vi "LogBuffer.vi"(0 "tdms file in":refnum<k34>, 1 "Buffer in":refnum<queue>, 5 "sizeOfBlock":i32, 7 "NumOfChannels":i32=65, 11 "error in (no error)":errorcluster, 12 "resetResample":bool, 13 "resample factor":cluster{"interpolation":i32, "decimation":i32}={"interpolation"=1, "decimation"=25}) -> (4 "tdms file out":refnum<k34>, 15 "error out":errorcluster)   [LabVIEW 2017, in "BufferLogging.lvlib"]
doc: "Log a single buffer. Decimate if configured."
uses:
  BufferLogging.lvlib
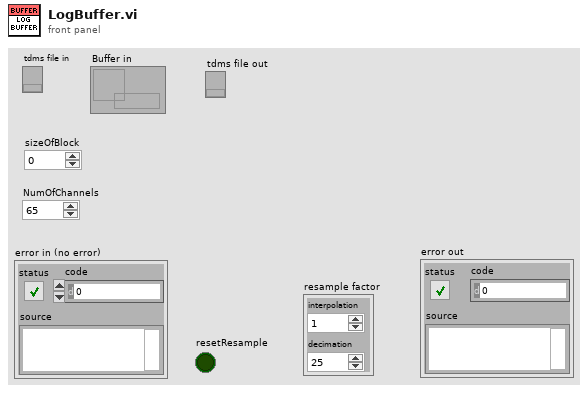
[diagram p1: front panel]
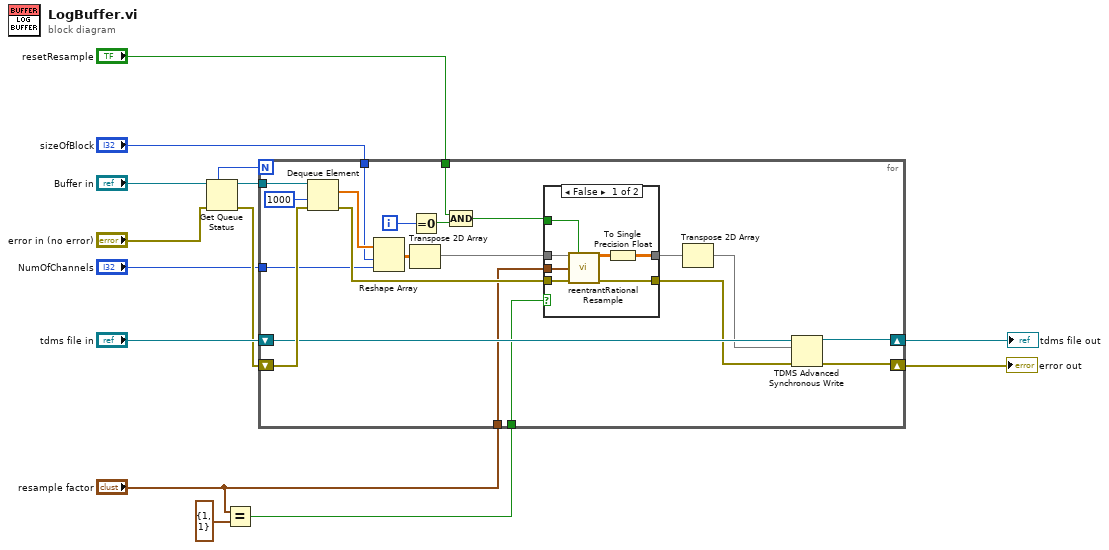
[diagram p0: block diagram]
diagram:
  n1 = Get Queue Status(queue="Buffer in", error in (no error)="error in (no error)") -> (queue out=w11:refnum<queue>, max queue size=w9:i32, error out=w8:errorcluster)  [unwired: 1 in, 5 out]
  n2 = Equal?(x="resample factor", y=cluster{"interpolation":i32, "decimation":i32} {"interpolation"=1, "decimation"=1}) -> (x = y?=w4:bool)
  n3 = for {
    N: w9 -> [_]
    tunnel: "sizeOfBlock" -> [w32]
    shift-right: [w26] -> w14
    shift-left: w8 -> [w35]
    tunnel: w11 -> [w29]
    shift-right: [w27] -> w13
    shift-left: "tdms file in" -> [w28]
    tunnel: "NumOfChannels" -> [w23]
    tunnel: "resetResample" -> [w21]
    tunnel: "resample factor" -> [w19]
    tunnel: w4 -> [w18]
    i -> [w31]
    n4 = Dequeue Element(queue=w29, timeout in ms (-1)=1000, error in (no error)=w35) -> (element=w33:sgl[], error out=w25:errorcluster)  [unwired: 2 out]
    n5 = Reshape Array(w33, w32, w23) -> (w30:sgl[][])
    n6 = Transpose 2D Array(2D array=w30) -> (transposed array=w24:sgl[][])
    n7 = Equal To 0?(x=w31) -> (x = 0?=w22:bool)
    n8 = Compound Arithmetic op=AND(w21, w22) -> (w20:bool)
    n9 = case shown="False" w18 {
      tunnel: [w36 w44] -> w16
      tunnel: w25 -> [w42 w43]
      tunnel: [w41 w43] -> w17
      tunnel: w24 -> [w40 w44]
      tunnel: w20 -> [w39 _]
      tunnel: w19 -> [w38 _]
      frame False {
        n10 = call "reentrantRationalResample.vi"("X"=w40, "reset"=w39, "resample factor"=w38, "error in (no error)"=w42) -> ("Y"=w37:dbl[][], "error out"=w41:errorcluster)  [unwired: 10 in]
        n11 = To Single Precision Float(number=w37) -> (single precision float=w36:sgl[][])
      }
      frame True {
      }
    }
    n12 = Transpose 2D Array(2D array=w16) -> (transposed array=w15:sgl[][])
    n13 = TDMS Advanced Synchronous Write(8:w17, 10:w15, 11:w28) -> (0:w26:errorcluster, 3:w27:refnum<k34>)
  }
  "error out" <- w14
  "tdms file out" <- w13
